vi "SVMAlphaBetaFXP_src.vi"(0 "alpha":fxp<+/-,32,4> caption="voltage alpha", 1 "max":fxp<+/-,32,4>=0.999969482421875 caption="max voltage", 5 "beta":fxp<+/-,32,4> caption="voltage beta") -> (4 "Upercent":fxp<+/-,32,4> caption="u voltage", 6 "Vpercent":fxp<+/-,32,4> caption="v voltage", 8 "Wpercent":fxp<+/-,32,4> caption="w voltage", 15 "Sector":u8)   [LabVIEW 2015]
panel:
  out "_s1":fxp<+/-,32,4> format="%.18g"
  out "_s2":fxp<+/-,32,4> format="%.16g"
  out "_s3":fxp<+/-,32,4> format="%.16g"
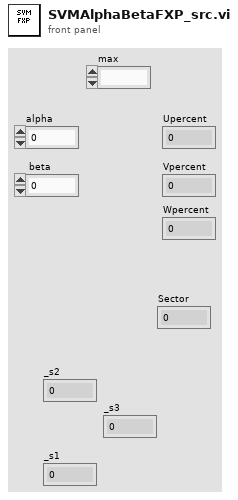
[diagram p1: front panel]
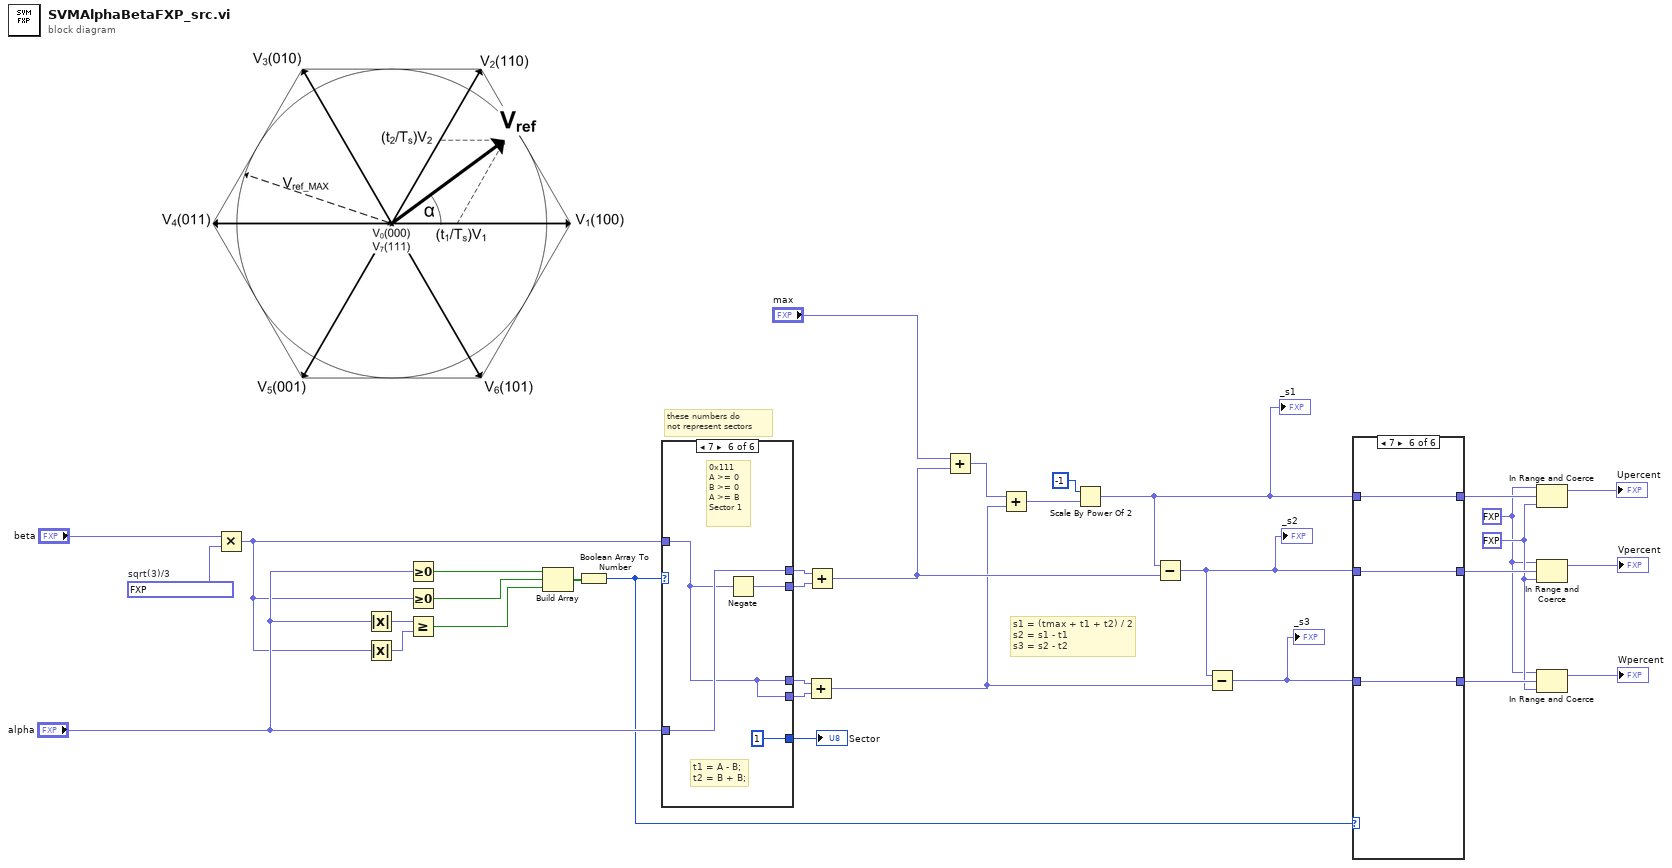
[diagram p0: block diagram]
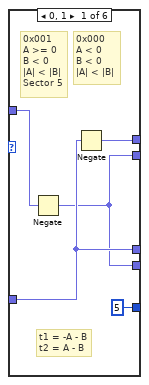
[diagram p2: hidden frame]
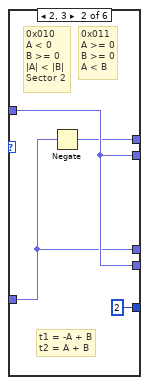
[diagram p3: hidden frame]
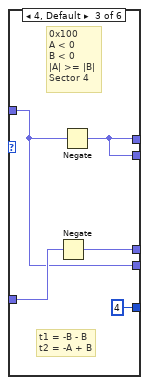
[diagram p4: hidden frame]
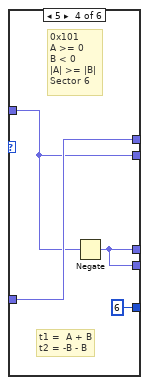
[diagram p5: hidden frame]
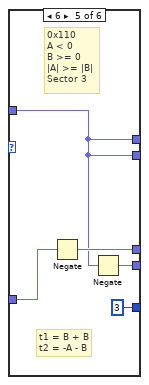
[diagram p6: hidden frame]
diagram:
  w13 = fxp<+,16,1> 0.577362060546875  # sqrt(3)/3
  w24 = fxp<+/-,32,4> 0.0 ("upper limit")
  w23 = fxp<+/-,32,4> 1.0 ("upper limit")
  # "s1 = (tmax + t1 + t2) / 2\ns2 = s1 - t1\ns3 = s2 - t2"
  # "these numbers do \nnot represent sectors"
  n1 = Multiply(x="beta", y=w13) -> (x*y=w14:fxp<+/-,32,4>)
  n2 = Absolute Value(x="alpha") -> (abs(x)=w12:fxp<+,32,4>)
  n3 = Absolute Value(x=w14) -> (abs(x)=w11:fxp<+,32,4>)
  n4 = Greater Or Equal To 0?(x="alpha") -> (x >= 0?=w9:bool)
  n5 = Greater Or Equal To 0?(x=w14) -> (x >= 0?=w8:bool)
  n6 = Greater Or Equal?(x=w12, y=w11) -> (x >= y?=w7:bool)
  n7 = Build Array(w9, w8, w7) -> (w10:bool[])
  n8 = Boolean Array To Number(Boolean array=w10) -> (number=w19:u8)
  n9 = case shown="7" w19 {
    tunnel: w14 -> [w38 w42 w44 w50 w54 w58]
    tunnel: "alpha" -> [w36 w40 w47 w51 w56 w59]
    tunnel: [w37 w41 w45 w51 w54 w59] -> w18
    tunnel: [w35 w42 w45 w50 w54 w60] -> w17
    tunnel: [w36 w40 w46 w49 w55 w58] -> w16
    tunnel: [w35 w42 w44 w49 w53 w58] -> w15
    tunnel: [u8 5 u8 2 u8 4 u8 6 u8 3 u8 1] -> w1
    frame 0, 1 {
      # "0x000\nA < 0\nB < 0\n|A| < |B|"
      # "t1 = -A - B\nt2 = A - B"
      # "0x001\nA >= 0\nB < 0\n|A| < |B|\nSector 5"
      n10 = Negate(x=w38) -> (-x=w35:fxp<+/-,33,5>)
      n11 = Negate(x=w36) -> (-x=w37:fxp<+/-,33,5>)
    }
    frame 2, 3 {
      # "0x011\nA >= 0\nB >= 0\nA < B"
      # "t1 = -A + B\nt2 = A + B"
      # "0x010\nA < 0\nB >= 0\n|A| < |B|\nSector 2"
      n12 = Negate(x=w40) -> (-x=w41:fxp<+/-,33,5>)
    }
    frame 4, Default {
      # "t1 = -B - B\nt2 = -A + B"
      # "0x100\nA < 0\nB < 0\n|A| >= |B|\nSector 4"
      n13 = Negate(x=w47) -> (-x=w46:fxp<+/-,33,5>)
      n14 = Negate(x=w44) -> (-x=w45:fxp<+/-,33,5>)
    }
    frame 5 {
      # "t1 =  A + B\nt2 = -B - B"
      # "0x101\nA >= 0\nB < 0\n|A| >= |B|\nSector 6"
      n15 = Negate(x=w50) -> (-x=w49:fxp<+/-,33,5>)
    }
    frame 6 {
      # "t1 = B + B\nt2 = -A - B"
      # "0x110\nA < 0\nB >= 0\n|A| >= |B|\nSector 3"
      n16 = Negate(x=w56) -> (-x=w55:fxp<+/-,33,5>)
      n17 = Negate(x=w54) -> (-x=w53:fxp<+/-,33,5>)
    }
    frame 7 {
      # "t1 = A - B;\nt2 = B + B;"
      # "0x111\nA >= 0\nB >= 0\nA >= B\nSector 1"
      n18 = Negate(x=w58) -> (-x=w60:fxp<+/-,16,1>)
    }
  }
  "Sector" <- w1
  n19 = Add(x=w16, y=w15) -> (x+y=w2:fxp<+/-,34,6>)
  n20 = Add(x=w18, y=w17) -> (x+y=w3:fxp<+/-,34,6>)
  n21 = Add(x="max", y=w3) -> (x+y=w6:fxp<+/-,34,6>)
  n22 = Add(x=w6, y=w2) -> (x+y=w4:fxp<+/-,32,4>)
  n23 = Scale By Power Of 2(n=-1 ("x"), x=w4) -> (x*2^n=w22:fxp<+/-,32,4>)
  "_s1" <- w22
  n24 = Subtract(x=w22, y=w3) -> (x-y=w21:fxp<+/-,32,4>)
  "_s2" <- w21
  n25 = Subtract(x=w21, y=w2) -> (x-y=w20:fxp<+/-,32,4>)
  "_s3" <- w20
  n26 = case shown="7" w19 {
    tunnel: w21 -> [w63 w66 w67 w70 w73 w77]
    tunnel: w22 -> [w62 w65 w68 w72 w74 w78]
    tunnel: w20 -> [w61 w64 w69 w71 w75 w76]
    tunnel: [w62 w64 w68 w70 w73 w76] -> w26
    tunnel: [w61 w65 w67 w71 w74 w77] -> w25
    tunnel: [w63 w66 w69 w72 w75 w78] -> w27
    frame 0, 1, Default {
    }
    frame 2, 3 {
    }
    frame 4 {
    }
    frame 5 {
    }
    frame 6 {
    }
    frame 7 {
    }
  }
  n27 = In Range and Coerce(upper limit=w23, x=w27, lower limit=w24) -> (coerced(x)=→"Upercent":fxp<+/-,32,4>)  [unwired: 1 out]
  n28 = In Range and Coerce(upper limit=w23, x=w25, lower limit=w24) -> (coerced(x)=→"Vpercent":fxp<+/-,32,4>)  [unwired: 1 out]
  n29 = In Range and Coerce(upper limit=w23, x=w26, lower limit=w24) -> (coerced(x)=→"Wpercent":fxp<+/-,32,4>)  [unwired: 1 out]
